vi "LJT4_init.vi"(9 "dev_id":T1, 10 "conn_type":T2(ring), 11 "dev_type":enum16{"LJM_dtANY", "LJM_dtT4"}(ring)=enum."LJM_dtT4") -> (0 "error out":errorcluster, 1 "DeviceType Out":i32, 2 "ConnectionType Out":i32, 3 "Handle Out":i32, 4 "SN":i32)   [LabVIEW 2019]
uses:
  enum_dev_id.ctl
panel:
  in  "STREAM_RESOLUTION_INDEX":i32
  in  "STREAM_SETTLING_US":i32
  in  "AIN_ALL_RANGE":dbl format="%.3f"
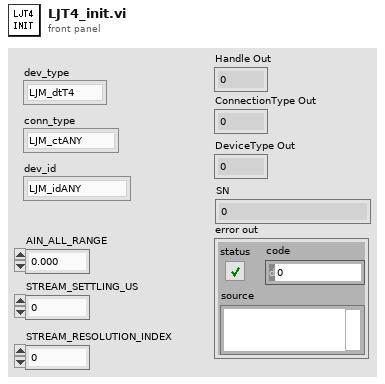
[diagram p1: front panel]
types:
  T1 = typedef "enum_dev_id.ctl" = enum16{"LJM_idANY", "192.168.24.185", "10.0.0.176", "440017305"}
  T2 = enum16{"LJM_ctANY", "LJM_ctUSB", "LJM_ctETHERNET"}
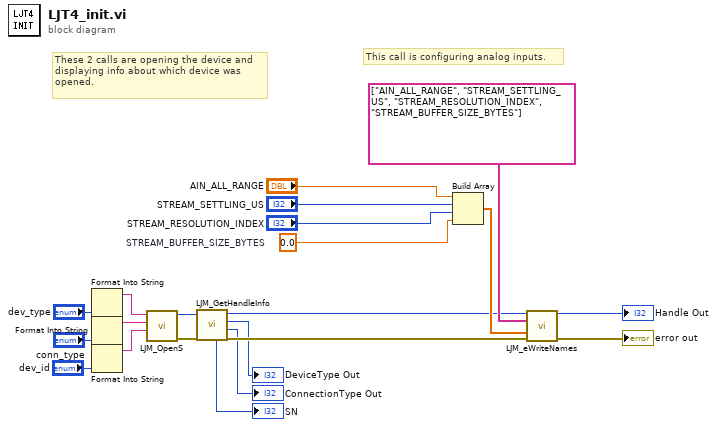
[diagram p0: block diagram]
diagram:
  w21 = 0.0  # STREAM_BUFFER_SIZE_BYTES
  # "This call is configuring analog inputs."
  # "These 2 calls are opening the device and\ndisplaying info about which device was\nopened."
  n1 = Format Into String("dev_type") -> (resulting string=w2:string)  [unwired: 3 in, 1 out]
  n2 = Format Into String("conn_type") -> (resulting string=w5:string)  [unwired: 3 in, 1 out]
  n3 = Format Into String("dev_id") -> (resulting string=w4:string)  [unwired: 3 in, 1 out]
  n4 = call "LJM_OpenS.vi"("Identifier"=w4, "ConnectionType"=w5, "DeviceType"=w2) -> ("error out"=w8:errorcluster, "Handle"=w9:i32)  [unwired: 7 in]
  n5 = call "LJM_GetHandleInfo.vi"("error in"=w8, "Handle In"=w9) -> ("error out"=w12:errorcluster, "ConnectionType"=→"ConnectionType Out":i32, "DeviceType"=→"DeviceType Out":i32, "Handle Out"=w13:i32, "SerialNumber"=→"SN":i32)  [unwired: 2 in, 3 out]
  n6 = Build Array("AIN_ALL_RANGE", "STREAM_SETTLING_US", "STREAM_RESOLUTION_INDEX", w21) -> (w18:dbl[])
  n7 = call "LJM_eWriteNames.vi"("Handle In"=w13, "aNames"=string[] ["AIN_ALL_RANGE", "STREAM_SETTLING_US", "STREAM_RESOLUTION_INDEX", "STREAM_BUFFER_SIZE_BYTES"], "aValuesIn"=w18, "error in"=w12) -> ("Handle Out"=→"Handle Out":i32, "error out"=→"error out":errorcluster)  [unwired: 9 in, 1 out]
